vi "Main_ver4.vi"() -> ()   [LabVIEW 2014]
uses:
  Program Files/National Instruments/LabVIEW 2014/examples/Instrument IO/Serial/support/Serial - Settings.ctl
  Program Files/National Instruments/LabVIEW 2014/examples/Instrument IO/Serial/support/Serial - XON-XOFF Characters.ctl
  Program Files/National Instruments/LabVIEW 2014/examples/Instrument IO/Serial/support/Serial - ASCII Characters.ctl
  <vilib>/Instr/_visa.llb/VISA Configure Serial Port (Instr).vi
panel:
  in  "REMOTE / MANUAL":bool=TRUE
  in  "RIGHT / LEFT":bool=TRUE
  in  "STEP TIME":dbl(slide)=1000.0 scale=100.0..2000.0
  in  "error IO":errorcluster
  in  "Termination Character":u8=13 format="%.0x"
  in  "End Write on Termination Character?":bool=TRUE
  in  "VISA resource name":refnum<visa-resource-name>="COM1"
  in  "XON/XOFF Characters":T1={"XON"=enum."DC1", "XOFF"=enum."DC3"}
  in  "Serial Settings":T3={"baud rate"=9600, "data bits"=8, "parity"=enum."None", "stop bits"=10, "flow control"=0} {"flow control" items=["None"=0, "XON/XOFF"=1, "RTS/CTS"=2, "DTR/DSR"=4]; "stop bits" items=["1.0"=10, "1.5"=15, "2.0"=20]; "data bits" min=5 max=8 step=1; "baud rate" items=["75"=75, "110"=110, "134"=134, "150"=150, "300"=300, "600"=600, "1200"=1200, "1800"=1800, "2400"=2400, "4800"=4800, "7200"=7200, "9600"=9600, "14400"=14400, "19200"=19200, "28800"=28800, "38400"=38400, "56000"=56000, "57600"=57600, "115200"=115200, "128000"=128000, "230400"=230400]}
  in  "End Read on Termination Character?":bool=TRUE
  out "Response":string
  in  "Read Count":u32=1000
  in  "Read":bool
  in  "Stop":bool
  in  "ON / OFF":bool=TRUE
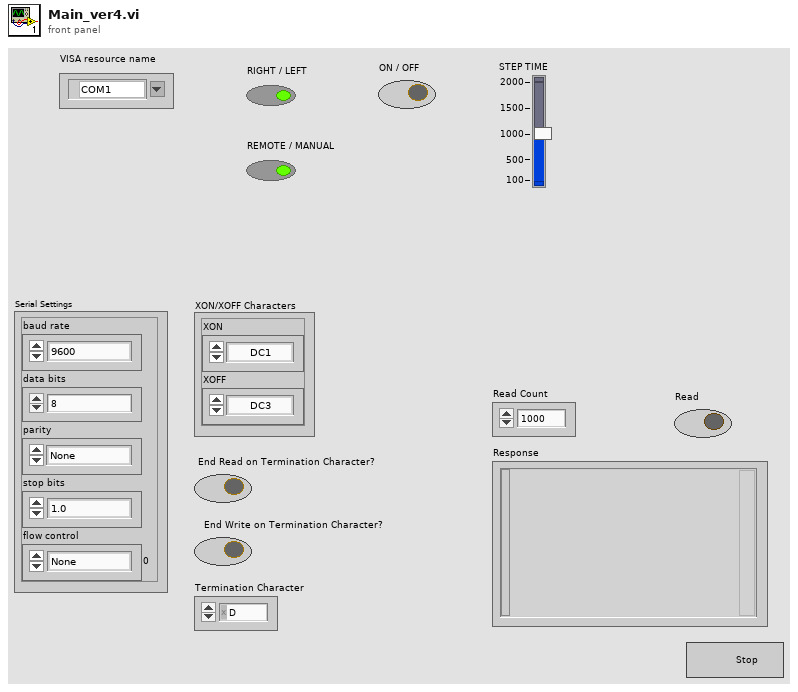
[diagram p1: front panel]
types:
  T1 = typedef "Serial - XON-XOFF Characters.ctl" = cluster{"XON":T2, "XOFF":T2}
  T2 = typedef "Serial - ASCII Characters.ctl" = enum16{"NUL", "SOH", "STX", "ETX", "EOT", "ENQ", "ACK", "BEL", "BS", "HT", "LF", "VT", "FF", "CR", "SO", "SI", "DLE", "DC1", "DC2", "DC3", "DC4", "NAK", "SYN", "ETB", "CAN", "EM", "SUB", "ESC", "FS", "GS", "RS", "US", "SP", "!", "\"", "#", "$", "%", "&", "'", "(", ")", "*", "+", ",", "- (-)", ".", "/", "0", "1", "2", "3", "4", "5", "6", "7", "8", "9", ":", ";", "<", "=", ">", "?", "@", "A", "B", "C", "D", "E", "F", "G", "H", "I", "J", "K", "L", "M", "N", "O", "P", "Q", "R", "S", "T", "U", "V", "W", "X", "Y", "Z", "[", "\\", "]", "^", "_", "`", "a", "b", "c", "d", "e", "f", "g", "h", "i", "j", "k", "l", "m", "n", "o", "p", "q", "r", "s", "t", "u", "v", "w", "x", "y", "z", "{", "|", "}", "~"}
  T3 = typedef "Serial - Settings.ctl" = cluster{"baud rate":u32, "data bits":u16, "parity":enum16{"None", "Odd", "Even", "Mark", "Space"}, "stop bits":u16, "flow control":u16}
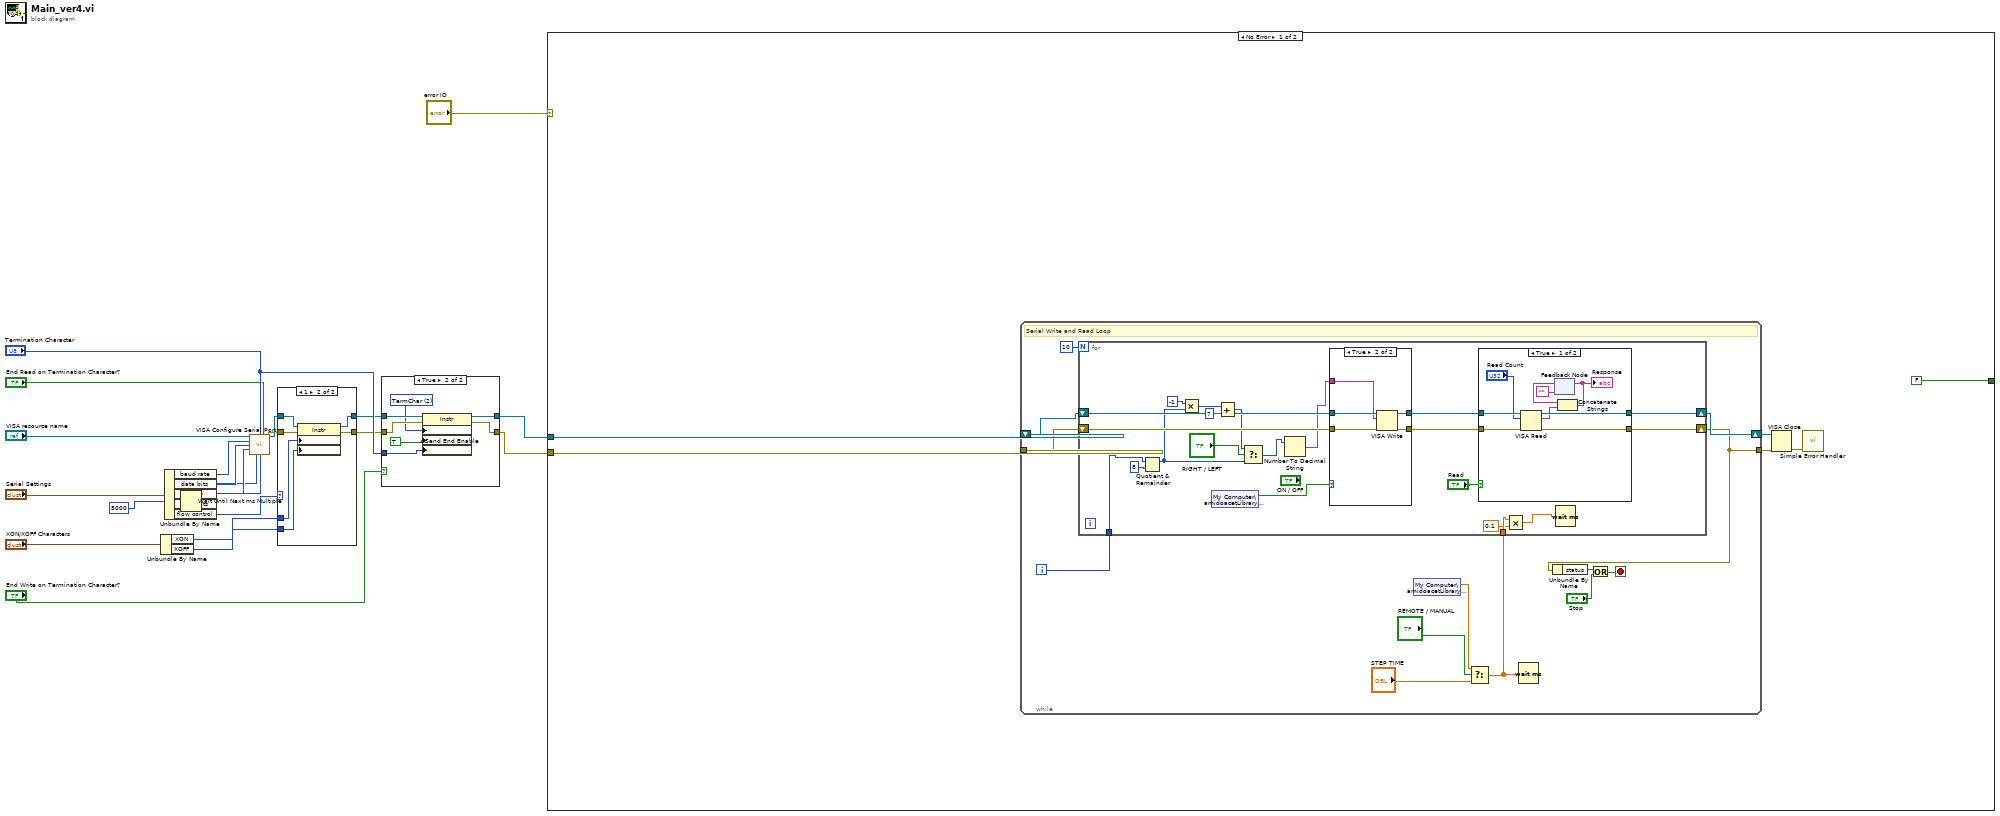
[diagram p0: block diagram]
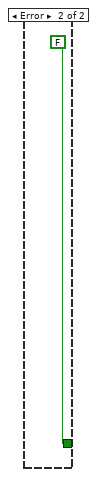
[diagram p6: hidden frame]
diagram:
  n1 = Unbundle By Name("XON/XOFF Characters") -> ("XON"=w16:T2, "XOFF"=w17:T2)
  n2 = Unbundle By Name("Serial Settings") -> ("baud rate"=w12:u32, "data bits"=w11:u16, "parity"=w10:enum16{"None", "Odd", "Even", "Mark", "Space"}, "stop bits"=w9:u16, "flow control"=w15:u16)
  n3 = Wait Until Next ms Multiple(millisecond multiple=u32 5000) -> ()  [unwired: 1 out]
  n4 = call-poly "VISA Configure Serial Port"("VISA resource name"="VISA resource name", "termination char\n(0xA = '\\n' = LF)"="Termination Character", "Enable Termination\nChar (T)"="End Read on Termination Character?", "baud rate (9600)"=w12, "data bits (8)"=w11, "parity (0:none)"=w10, "stop bits (10: 1 bit)"=w9, "flow control (0:none)"=w15) -> ("VISA resource name out"=w8:refnum<visa-resource-name>, "error out"=w7:errorcluster)  [unwired: 2 in, 4 out]
  n5 = case shown="1" w15 {
    tunnel: [w22 w29] -> w18
    tunnel: [w23 w28] -> w19
    tunnel: w7 -> [w22 w27]
    tunnel: w8 -> [w23 w26]
    tunnel: w16 -> [_ w25]
    tunnel: w17 -> [_ w24]
    frame Default {
    }
    frame 1 {
      n6 = property class="Instr"(reference=w26, error in=w27, "Serial Settings:Flow Control XON Character"=w25, "Serial Settings:Flow Control XOFF Character"=w24) -> (reference out=w28:refnum<visa-resource-name>, error out=w29:errorcluster)
    }
  }
  n7 = case shown="True" "End Write on Termination Character?" {
    tunnel: w19 -> [w30 w38]
    tunnel: w18 -> [w31 w37]
    tunnel: [w30 w36] -> w3
    tunnel: [w31 w35] -> w2
    tunnel: "Termination Character" -> [_ w33]
    frame False {
    }
    frame True {
      w34 = u16 2 items=["None", "LastBit", "TermChar", "Break"] ("Serial Settings:Serial End Mode for Writes")
      n8 = property class="Instr"(reference=w38, error in=w37, "Serial Settings:End Mode for Writes"=w34, "Message Based Settings:Send End Enable"=TRUE, "Message Based Settings:Termination Character"=w33) -> (reference out=w36:refnum<visa-resource-name>, error out=w35:errorcluster)
    }
  }
  n9 = case shown="No Error" "error IO" {
    tunnel: [FALSE FALSE] -> _
    tunnel: w3 -> [w43 _]
    tunnel: w2 -> [w42 _]
    frame No Error {
      n10 = while {
        shift-right: [w57] -> w40
        shift-left: w43 -> [w47]
        tunnel: w42 -> [w56]
        tunnel: [w52] -> w39
        i -> [w48]
        stop <- w54 stop-if-true
        # "Serial Write and Read Loop"
        n11 = shared-variable "My Computer\\amidoacetLibrary.lvlib\\steps"() -> (w50:dbl)  [unwired: 1 in, 1 out]
        n12 = Select(t=w50, s="REMOTE / MANUAL", f="STEP TIME") -> (s? t:f=w45:dbl)
        n13 = for {
          N: 10 -> [_]
          shift-right: [w78] -> w57
          shift-left: w47 -> [w77]
          shift-right: [w72] -> w52
          shift-left: w56 -> [w76]
          tunnel: w48 -> [w62]
          tunnel: w45 -> [w60]
          n14 = Quotient & Remainder(x=w62, y=8) -> (x-y*floor(x/y)=w70:i32)  [unwired: 1 out]
          n15 = Multiply(x=-1, y=w70) -> (x*y=w66:i32)
          n16 = shared-variable "My Computer\\amidoacetLibrary.lvlib\\STOP"() -> (w58:bool)  [unwired: 1 in, 1 out]
          n17 = Add(x=w66, y=7) -> (x+y=w69:i32)
          n18 = Select(t=w69, s="RIGHT / LEFT", f=w70) -> (s? t:f=w63:i32)
          n19 = Number To Decimal String(number=w63) -> (decimal integer string=w71:string)  [unwired: 1 in]
          n20 = case shown="True" w58 {
            tunnel: w77 -> [w80 w85]
            tunnel: w76 -> [w79 w84]
            tunnel: [w80 w83] -> w75
            tunnel: [w79 w82] -> w74
            tunnel: w71 -> [_ w81]
            frame False {
            }
            frame True {
              n21 = VISA Write(VISA resource name=w85, write buffer=w81, error in (no error)=w84) -> (VISA resource name out=w83:refnum<visa-resource-name>, error out=w82:errorcluster)  [unwired: 1 out]
            }
          }
          n22 = case shown="True" "Read" {
            tunnel: [w92 w96] -> w78
            tunnel: w75 -> [w94 w96]
            tunnel: [w90 w95] -> w72
            tunnel: w74 -> [w93 w95]
            frame True {
              n23 = VISA Read(VISA resource name=w94, byte count="Read Count", error in (no error)=w93) -> (VISA resource name out=w92:refnum<visa-resource-name>, read buffer=w89:string, error out=w90:errorcluster)  [unwired: 1 out]
              n24 = feedback #1("") -> (w88:string)
              n25 = Concatenate Strings(w88, w89) -> (w87:string)
              "Response" <- w87
              n26 = feedback-in #1(w87) -> ()
            }
            frame False {
            }
          }
          n27 = Multiply(x=w60, y=0.1) -> (x*y=w61:dbl)
          n28 = Wait (ms)(milliseconds to wait=w61) -> ()  [unwired: 1 out]
        }
        n29 = Wait (ms)(milliseconds to wait=w45) -> ()  [unwired: 1 out]
        n30 = Unbundle By Name(w52) -> ("status"=w55:bool)
        n31 = Or(x=w55, y="Stop") -> (x .or. y?=w54:bool)
      }
      n32 = VISA Close(VISA resource name=w40, error in (no error)=w39) -> (error out=w41:errorcluster)
      n33 = call <vilib>:"Simple Error Handler.vi"("error in (no error)"=w41) -> ()  [unwired: 1 in, 8 out]
    }
    frame Error {
    }
  }
